vi "XW_Linearise_+_temp_comp_PN.vi"(5 "Calib const":dbl[](array[numeric]) format="%.4f", 6 "XW2 voltage":dbl[](array[numeric]) format="%.4f", 7 "XW1 voltage":dbl[](array[numeric]) format="%.4f") -> (0 "U1":dbl[](array[numeric]) format="%.2f", 1 "V":dbl[](array[numeric]) format="%.2f", 2 "U2":dbl[](array[numeric]) format="%.2f", 3 "U":dbl[](array[numeric]) format="%.2f")   [LabVIEW 2010]
uses:
  Globals/Meas_global.vi
  XW calib map/XW_Map_Global.vi
panel:
  out "no. of pts outside map":i32
  # "(for trimesh only):"
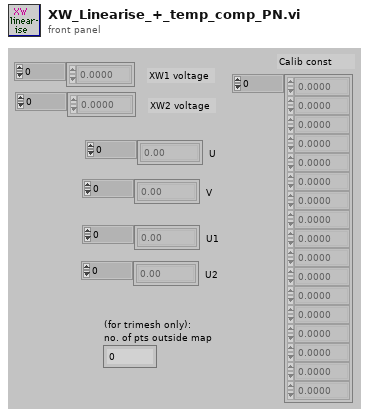
[diagram p1: front panel]
types:
  T1 = typedef "Map method.ctl" = enum16{"Triangle mesh", "Polynomial surface", "Const. Psi_eff (std.)", "Psi_eff = f(Umagn.)", "Psi_eff, k = f(Umagn.)"}
  T2 = cluster{"Calib const[0]":dbl, "Calib const[1]":dbl, "Calib const[2]":dbl, "Calib const[3]":dbl, "Calib const[4]":dbl, "Calib const[5]":dbl, "Calib const[6]":dbl, "Calib const[7]":dbl, "Calib const[8]":dbl, "Calib const[9]":dbl, "Calib const[10]":dbl, "Calib const[11]":dbl, "Calib const[12]":dbl, "Calib const[13]":dbl, "Calib const[14]":dbl, "Calib const[15]":dbl, "Calib const[16]":dbl, "Calib const[17]":dbl}
  T3 = typedef "Trimmed down TreeNode2D.ctl" = cluster{"Xmax":dbl, "Xmin":dbl, "Ymax":dbl, "Ymin":dbl, "Xc":dbl, "Yc":dbl, "ObjIndexList":i32[], "NodeQ1Index":i32, "NodeQ2Index":i32, "NodeQ3Index":i32, "NodeQ4Index":i32}
  T4 = typedef "Triangle2D.ctl" = cluster{"V10":dbl[], "V20":dbl[], "1/det":dbl, "V0":cluster{"PosVector":dbl[], "ValueVector":dbl[]}, "V1":cluster{"PosVector":dbl[], "ValueVector":dbl[]}, "V2":cluster{"PosVector":dbl[], "ValueVector":dbl[]}, "V21":dbl[]}
  T5 = enum16{"2nd component as calculated", "2nd component multipled by -1"}
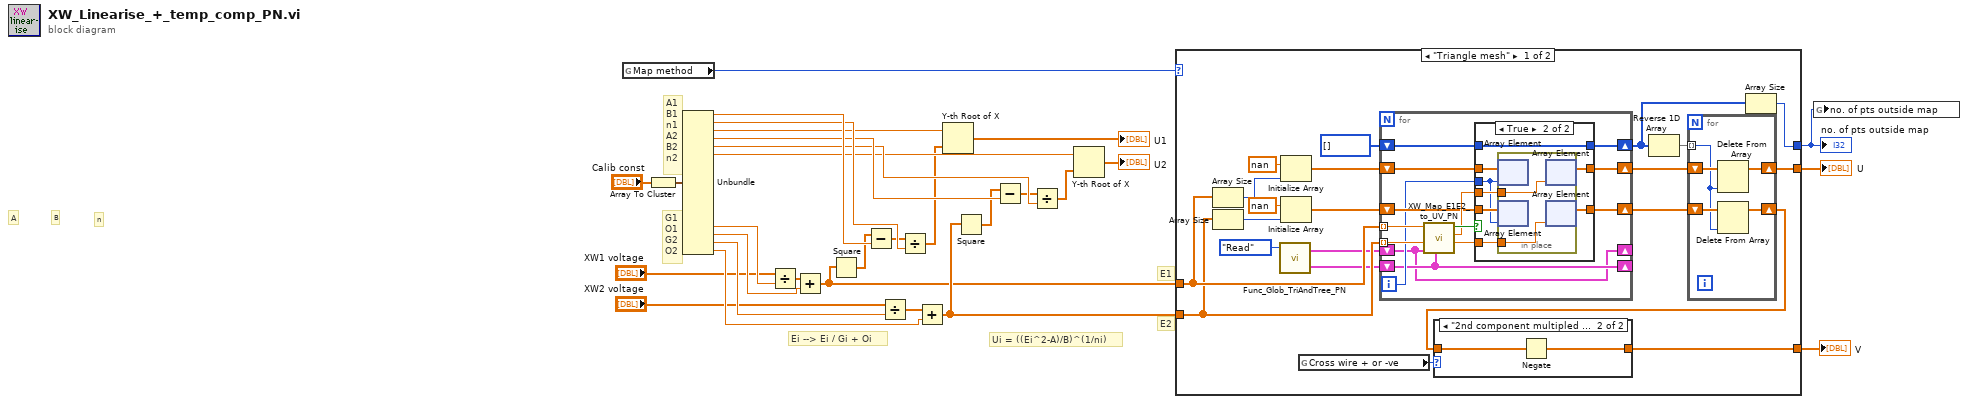
[diagram p0: block diagram]
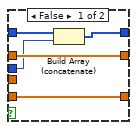
[diagram p2: hidden frame]
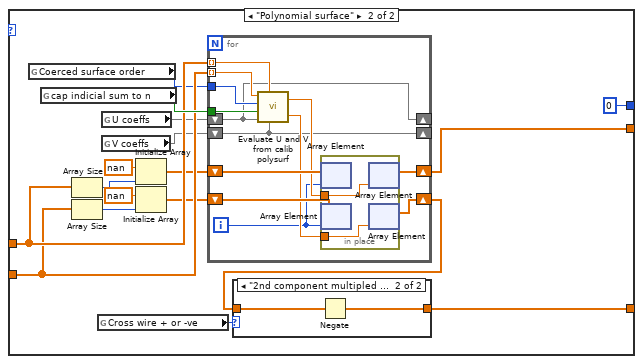
[diagram p4: hidden frame]
diagram:
  # "E2"
  # "E1"
  # "Ui = ((Ei^2-A)/B)^(1/ni)"
  # "Ei --> Ei / Gi + Oi"
  # "G1\nO1\nG2\nO2"
  # "A1\nB1\nn1\nA2\nB2\nn2"
  # "n"
  # "B"
  # "A"
  n1 = global read "XW_Map_Global.vi" "Map method"() -> (w2:T1)
  n2 = Array To Cluster(array="Calib const") -> (cluster=w30:T2)
  n3 = Unbundle(w30) -> ("Calib const[0]"=w24:dbl, "Calib const[1]"=w23:dbl, "Calib const[2]"=w22:dbl, "Calib const[3]"=w21:dbl, "Calib const[4]"=w20:dbl, "Calib const[5]"=w19:dbl, "Calib const[14]"=w29:dbl, "Calib const[15]"=w28:dbl, "Calib const[16]"=w27:dbl, "Calib const[17]"=w26:dbl)  [unwired: 8 out]
  n4 = Divide(x="XW1 voltage", y=w29) -> (x/y=w9:dbl[])
  n5 = Add(x=w9, y=w28) -> (x+y=w5:dbl[])
  n6 = Square(x=w5) -> (x^2=w11:dbl[])
  n7 = Subtract(x=w11, y=w24) -> (x-y=w12:dbl[])
  n8 = Divide(x="XW2 voltage", y=w27) -> (x/y=w10:dbl[])
  n9 = Divide(x=w12, y=w23) -> (x/y=w13:dbl[])
  n10 = Add(x=w10, y=w26) -> (x+y=w6:dbl[])
  n11 = Y-th Root of X(1:w13, 2:w22) -> (0:→"U1":dbl[])
  n12 = Square(x=w6) -> (x^2=w16:dbl[])
  n13 = Subtract(x=w16, y=w21) -> (x-y=w14:dbl[])
  n14 = Divide(x=w14, y=w20) -> (x/y=w15:dbl[])
  n15 = Y-th Root of X(1:w15, 2:w19) -> (0:→"U2":dbl[])
  n16 = case shown="\"Triangle mesh\"" w2 {
    tunnel: w6 -> [w45 w97]
    tunnel: w5 -> [w47 w98]
    tunnel: [w36 w94] -> w4
    tunnel: [w51 w105] -> w3
    tunnel: [w35 0] -> w1
    frame "Triangle mesh" {
      n17 = Array Size(array=w47) -> (size(s)=w46:i32)
      n18 = Array Size(array=w45) -> (size(s)=w44:i32)
      n19 = call "Func_Glob_TriAndTree_PN.vi"("Action"=enum16{"Read", "Write"}."Read") -> ("Trimmed down TreeNode array OUT"=w31:T3[], "Corrected triangles OUT"=w32:T4[])  [unwired: 2 in]
      n20 = Initialize Array(nan ("element"), w46) -> (w42:dbl[])
      n21 = Initialize Array(nan ("element"), w44) -> (w43:dbl[])
      n22 = global read "Meas_global.vi" "Cross wire + or -ve"() -> (w50:T5)
      n23 = for {
        tunnel: w47 -> [w70] mode=indexing
        tunnel: w45 -> [w69] mode=indexing
        shift-right: [w58] -> w34
        shift-left: i32[] [] -> [w57]
        shift-right: [w65] -> w40
        shift-left: w42 -> [w64]
        shift-right: [w62] -> w39
        shift-left: w43 -> [w63]
        shift-right: [w59] -> _
        shift-left: w32 -> [w59]
        shift-right: [w60] -> _
        shift-left: w31 -> [w60]
        i -> [w61]
        n24 = call "XW_Map_E1E2_to_UV_PN.vi"("Trimmed down TreeNode array"=w60, "Triangulated XW Calib Map Mesh"=w59, "(E2 / G2) + O2 (Volts)"=w69, "(E1 / G1) + O1 (Volts)"=w70) -> ("V (m/s)"=w66:dbl, "U (m/s)"=w67:dbl, "Voltages are inside calibrated region"=w68:bool)  [unwired: 5 out]
        n25 = case shown="True" w68 {
          tunnel: w67 -> [_ w79]
          tunnel: w57 -> [w71 w83]
          tunnel: [w72 w83] -> w58
          tunnel: w66 -> [_ w78]
          tunnel: [w75 w81] -> w65
          tunnel: w64 -> [w75 w82]
          tunnel: w63 -> [w74 w80]
          tunnel: [w74 w77] -> w62
          tunnel: w61 -> [w73 w76]
          frame False {
            n26 = Build Array (concatenate)(w71, w73) -> (w72:i32[])
          }
          frame True {
            n27 = in-place {
              in-place-border: w79 -> [w85]
              in-place-border: w78 -> [w84]
              n28 = in-place-array #1(w82, w76) -> ()  [unwired: 1 out]
              n29 = in-place-array #2(w80, w76) -> ()  [unwired: 1 out]
              n30 = in-place-array #1(w85) -> (w81:dbl[])  [unwired: 1 out]
              n31 = in-place-array #2(w84) -> (w77:dbl[])  [unwired: 1 out]
            }
          }
        }
      }
      n32 = Reverse 1D Array(array=w34) -> (reversed array=w38:i32[])
      n33 = for {
        shift-right: [w53] -> w36
        shift-left: w40 -> [w56]
        shift-right: [w54] -> w37
        shift-left: w39 -> [w55]
        tunnel: w38 -> [w52] mode=indexing
        n34 = Delete From Array(array=w56, index=w52) -> (array with subset deleted=w53:dbl[])  [unwired: 1 in, 1 out]
        n35 = Delete From Array(array=w55, index=w52) -> (array with subset deleted=w54:dbl[])  [unwired: 1 in, 1 out]
      }
      n36 = case shown="\"2nd component multipled by -1\"" w50 {
        tunnel: [w86 w88] -> w51
        tunnel: w37 -> [w86 w87]
        frame "2nd component as calculated" {
        }
        frame "2nd component multipled by -1" {
          n37 = Negate(x=w87) -> (-x=w88:dbl[])
        }
      }
      n38 = Array Size(array=w34) -> (size(s)=w35:i32)
    }
    frame "Polynomial surface" {
      n39 = global read "XW_Map_Global.vi" "Coerced surface order"() -> (w92:i32)
      n40 = global read "XW_Map_Global.vi" "cap indicial sum to n"() -> (w103:bool)
      n41 = Array Size(array=w98) -> (size(s)=w100:i32)
      n42 = Array Size(array=w97) -> (size(s)=w99:i32)
      n43 = global read "Meas_global.vi" "Cross wire + or -ve"() -> (w104:T5)
      n44 = global read "XW_Map_Global.vi" "U coeffs"() -> (w91)
      n45 = global read "XW_Map_Global.vi" "V coeffs"() -> (w90)
      n46 = Initialize Array(nan ("element"), w100) -> (w96:dbl[])
      n47 = Initialize Array(nan ("element"), w99) -> (w95:dbl[])
      n48 = for {
        tunnel: w98 -> [w118] mode=indexing
        tunnel: w97 -> [w117] mode=indexing
        tunnel: w103 -> [w116]
        shift-right: [w114] -> w93
        shift-left: w95 -> [w112]
        shift-right: [w115] -> w94
        shift-left: w96 -> [w113]
        tunnel: w92 -> [w108]
        shift-right: [w107] -> _
        shift-left: w90 -> [w107]
        shift-right: [w106] -> _
        shift-left: w91 -> [w106]
        i -> [w109]
        n49 = call "Evaluate U and V from calib polysurf.vi"("alpha(rad) coeffs"=w107, "E1 / G1 + O1"=w118, "Ucal coeffs"=w106, "cap indicial sum to n"=w116, "surface order (n)"=w108, "E2 / G2 + O2"=w117) -> ("V (m/s)"=w111:dbl, "U (m/s)"=w110:dbl)
        n50 = in-place {
          in-place-border: w110 -> [w120]
          in-place-border: w111 -> [w119]
          n51 = in-place-array #3(w113, w109) -> ()  [unwired: 1 out]
          n52 = in-place-array #4(w112, w109) -> ()  [unwired: 1 out]
          n53 = in-place-array #3(w120) -> (w115:dbl[])  [unwired: 1 out]
          n54 = in-place-array #4(w119) -> (w114:dbl[])  [unwired: 1 out]
        }
      }
      n55 = case shown="\"2nd component multipled by -1\"" w104 {
        tunnel: [w121 w123] -> w105
        tunnel: w93 -> [w121 w122]
        frame "2nd component as calculated" {
        }
        frame "2nd component multipled by -1" {
          n56 = Negate(x=w122) -> (-x=w123:dbl[])
        }
      }
    }
  }
  "U" <- w4
  "V" <- w3
  "no. of pts outside map" <- w1
  n57 = global write "XW_Map_Global.vi" "no. of pts outside map"(w1) -> ()
